vi "Teleop.vi"(10 "Match Info":T1={"Autonomous Elapsed Seconds"=0.0, "TeleOp Elapsed Seconds"=0.0, "Disabled Elapsed Seconds"=0.0, "Visited Autonomous"=FALSE, "Visited TeleOp"=FALSE, "Visited Disabled"=FALSE, "Autonomous Settings"={"Autonomous Style"=enum."Independent", "VI Refnum"=refnum}}, 11 "Call Context":T2) -> ()   [LabVIEW 2013]
doc: "This VI is called for each TeleOp packet received from the DS where the robot is not disabled. It is often used to read from the joysticks and update I/O or to update setpoints for timed control loops. It should complete and return within 20 milliseconds or it may miss DS packets."
uses:
  <vilib>/Rock Robotics/WPI/DriverStation/WPI_DriverStationDerivedRobotMode.ctl
  <vilib>/Rock Robotics/WPI/DriverStation/WPI_DriverStationMatch Info.ctl
  <vilib>/Rock Robotics/WPI/Solenoid/WPI_SolenoidValue.ctl
  Robot Global Data.vi
  <vilib>/Rock Robotics/WPI/Joystick/WPI_JoystickGetSetRefNum.vi
panel:
  in  "Xbox Controller?":bool
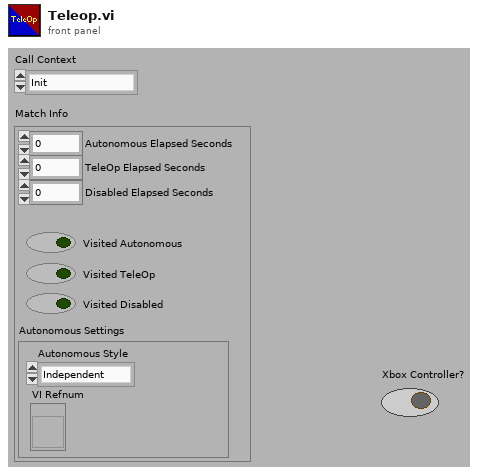
[diagram p1: front panel]
types:
  T1 = typedef "WPI_DriverStationMatch Info.ctl" = cluster{"Autonomous Elapsed Seconds":dbl, "TeleOp Elapsed Seconds":dbl, "Disabled Elapsed Seconds":dbl, "Visited Autonomous":bool, "Visited TeleOp":bool, "Visited Disabled":bool, "Autonomous Settings":cluster{"Autonomous Style":enum16{"Iterative", "Independent"}, "VI Refnum":refnum<vi>}}
  T2 = typedef "WPI_DriverStationDerivedRobotMode.ctl" = enum16{"Init", "Execute", "Stop"}
  T3 = typedef "WPI_SolenoidValue.ctl" = enum16{"Off", "On", "Forward", "Reverse"}
  T4 = typedef "WPI_JoystickDevRef.ctl" = cluster{"Device":T5}
  T5 = typedef "WPI_JoystickDeviceEnum.ctl" = enum16{"USB 1", "USB 2", "USB 3", "USB 4", "Kinect 1", "Kinect 2"}
  T6 = cluster{"axis 1 (x)":dbl, "axis 2 (y)":dbl, "axis 3 (throttle)":dbl, "axis 4":dbl, "axis 5":dbl, "axis 6":dbl}
  T7 = typedef "WPI_JoystickButtonState.ctl" = cluster{"Button 1":bool, "Button 2":bool, "Button 3":bool, "Button 4":bool, "Button 5":bool, "Button 6":bool, "Button 7":bool, "Button 8":bool, "Button 9":bool, "Button 10":bool, "Button 11":bool, "Button 12":bool}
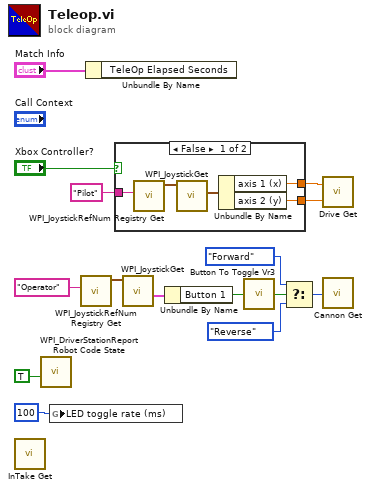
[diagram p0: block diagram]
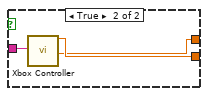
[diagram p2: hidden frame]
diagram:
  n1 = call "InTake Get.vi"() -> ()  [unwired: 3 in]
  n2 = call <vilib>:"WPI_DriverStationReport Robot Code State.vi"("TeleOp"=TRUE ("Autonomous")) -> ()  [unwired: 10 in, 1 out]
  n3 = global write "Robot Global Data.vi" "LED toggle rate (ms)"(u32 100 ("LED ms toggle rate")) -> ()
  n4 = call <vilib>:"WPI_JoystickRefNum Registry Get.vi"("refnum name"="Operator") -> ("JoystickDevRef"=w8:T4)  [unwired: 9 in, 1 out]
  n5 = Unbundle By Name("Match Info") -> ()  [unwired: 1 out]
  n6 = case shown="False" "Xbox Controller?" {
    tunnel: "Pilot" ("refnum name") -> [w19 w23]
    tunnel: [w17 w22] -> w10
    tunnel: [w16 w21] -> w9
    frame False {
      n7 = call <vilib>:"WPI_JoystickRefNum Registry Get.vi"("refnum name"=w19) -> ("JoystickDevRef"=w20:T4)  [unwired: 9 in, 1 out]
      n8 = call <vilib>:"WPI_JoystickGet.vi"("JoystickDevRef"=w20) -> ("Axes"=w18:T6)  [unwired: 4 in, 2 out]
      n9 = Unbundle By Name(w18) -> ("axis 1 (x)"=w16:dbl, "axis 2 (y)"=w17:dbl)
    }
    frame True {
      n10 = call "Xbox Controller.vi"("Joystick Name"=w23) -> ("Left Stick Y"=w22:dbl, "Right Stick Y"=w21:dbl)  [unwired: 3 in, 14 out]
    }
  }
  n11 = call <vilib>:"WPI_JoystickGet.vi"("JoystickDevRef"=w8) -> ("Buttons"=w6:T7)  [unwired: 4 in, 2 out]
  n12 = Unbundle By Name(w6) -> ("Button 1"=w5:bool)
  n13 = call "Button To Toggle Vr3.vi"("InValue"=w5) -> ("Result"=w3:bool)
  n14 = Select(t=WPI_SolenoidValue."Forward" ("Shoot!"), s=w3, f=WPI_SolenoidValue."Reverse" ("Shoot!")) -> (s? t:f=w1:T3)
  n15 = call "Drive Get.vi"("Y"=w10, "X"=w9) -> ()  [unwired: 1 in]
  n16 = call "Cannon Get.vi"("Shoot!"=w1) -> ()
